vi "Global X Border.vi"() -> ()   [LabVIEW 2014]
panel:
  out "GlobalXBorder":dbl=10.0
  # "GlobalXBorder is the amount of extra space on the field compared to ACTUAL \nfield as Intensity Graph. So if Global FieldLengthX = 100, then the  bottom rightmost corner is\nat x-coordinate 110 if GlobalXBorder is 10"
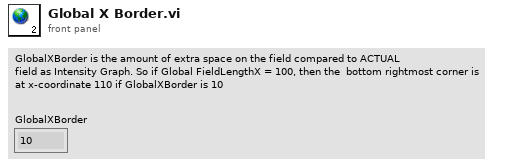
[diagram p1: front panel]
diagram:
